vi "open log file directory.vi"   [LabVIEW 2020]
uses:
  <vilib>/Utility/sysdir.llb/System Directory Type.ctl
types:
  T1 = typedef "System Directory Type.ctl" = i32
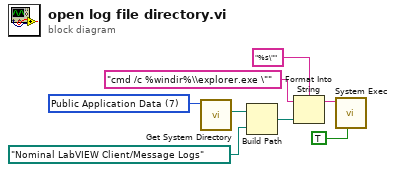
[diagram p0: block diagram]
diagram:
  w8 = T1 7 items=["User Home"=0, "User Desktop"=1, "User Documents"=2, "User Application Data"=3, "User Preferences"=4, "User Temporary"=5, "Public Documents"=6, "Public Application Data"=7, "Public Preferences"=8, "Public Cache"=13, "System Core Libraries"=9, "System Installed Libraries"=10, "Application Files"=11, "Boot Volume Root"=12] ("system directory type")
  n1 = call <vilib>:"Get System Directory.vi"("system directory type"=w8) -> ("system directory"=w7:path)  [unwired: 10 in]
  n2 = Build Path(base path=w7, name or relative path=path "Nominal LabVIEW Client/Message Logs") -> (appended path=w5:path)
  n3 = Format Into String(format string="%s\"" ("command line"), initial string="cmd /c %windir%\\explorer.exe \"" ("command line"), w5) -> (resulting string=w4:string)  [unwired: 1 in, 1 out]
  n4 = call <vilib>:"System Exec.vi"("run minimized? (F)"=TRUE, "command line"=w4) -> ()  [unwired: 6 in, 4 out]
